vi "TSM Relay Initialize Sessions.vi"(0 "TSM context":T1) -> (15 "error out":errorcluster)   [LabVIEW 2020]
doc: "Use this VI to initialize sessions for all NI 2567 Relay Driver Instruments in the pin map associated with the test program."
uses:
  <vilib>/NI_TestStand_SemiconductorModule/NI_TestStand_Semiconductor_Module.lvlibp/PinMap/General/SemiconductorModuleContext.ctl
  <instrlib>/niSwitch/niSwitch.llb/niSwitch Topologies.ctl
  <vilib>/NI_TestStand_SemiconductorModule/NI_TestStand_Semiconductor_Module.lvlibp
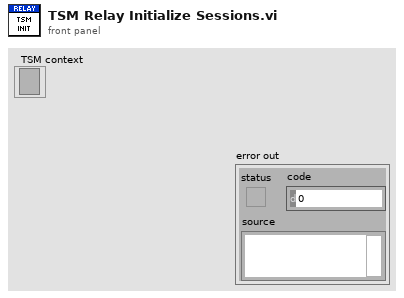
[diagram p1: front panel]
types:
  T1 = typedef "NI_TestStand_Semiconductor_Module.lvlibp/SemiconductorModuleContext.ctl" = refnum<k7>
  T2 = typedef "niSwitch Topologies.ctl" = string
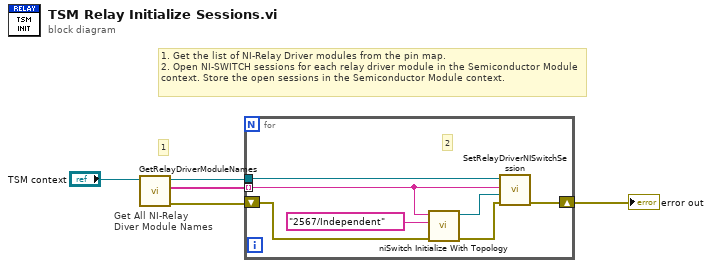
[diagram p0: block diagram]
diagram:
  # "1"
  # "1. Get the list of NI-Relay Driver modules from the pin map.\n2. Open NI-SWITCH sessions for each relay driver module in the Semiconductor Module context. Store the open sessions in the Semiconductor Module context."
  # "Get All NI-Relay\nDiver Module Names"
  n1 = call <vilib>:"GetRelayDriverModuleNames.vi"("Semiconductor Module Context"="TSM context") -> ("error out"=w1:errorcluster, "Module Names"=w2:string[], "Semiconductor Module Context Out"=w3:T1)  [unwired: 8 in]
  n2 = for {
    tunnel: w2 -> [w7] mode=indexing
    shift-right: [w11] -> w5
    shift-left: w1 -> [w8]
    tunnel: w3 -> [w12]
    # "2"
    n3 = call <instrlib>:"niSwitch Initialize With Topology.vi"("error in (no error)"=w8, "topology name"=T2 "2567/Independent", "resource name"=w7) -> ("error out"=w10:errorcluster, "instrument handle out"=w9:refnum<k15>)  [unwired: 7 in]
    n4 = call <vilib>:"SetRelayDriverNISwitchSession.vi"("error in (no error)"=w10, "NI-SWITCH Session"=w9, "Relay Driver Module Name"=w7, "Semiconductor Module Context"=w12) -> ("error out"=w11:errorcluster)  [unwired: 6 in, 1 out]
  }
  "error out" <- w5
